vi "ActFollowTrajectoryCommon.vi"(10 "Trajectory":T4 {"States"."POSE"."ROTATION"."SIN" format="%13.4f"; "States"."POSE"."ROTATION"."COS" format="%13.4f"; "States"."POSE"."ROTATION"."VALUE" format="%13.4f"; "States"."POSE"."TRANSLATION"."Y" format="%14.3f"; "States"."POSE"."TRANSLATION"."X" format="%14.3f"; "TotalTImeSecs" format="%20.3f"}, 11 "FirstTime":bool) -> (0 "Done":bool, 1 "AngularSpeedDmd":dbl, 2 "YSpeedDmd":dbl, 3 "XSpeedDmd":dbl)   [LabVIEW 2020]
uses:
  <vilib>/Rock Robotics/WPI/ThirdParty/JAS_Junk/TrajLib/Trajectory_Library.lvlib
  <vilib>/Rock Robotics/WPI/ThirdParty/JAS_Junk/TrajLib/TypeDef/TRANSLATION2D.ctl
  <vilib>/Rock Robotics/WPI/ThirdParty/JAS_Junk/TrajLib/TypeDef/ROTATION2D.ctl
  <vilib>/Rock Robotics/WPI/ThirdParty/JAS_Junk/TrajLib/TypeDef/POSE2D.ctl
  <vilib>/Rock Robotics/WPI/ThirdParty/JAS_Junk/TrajLib/TypeDef/TRAJ_STATE.ctl
  <vilib>/Rock Robotics/WPI/ThirdParty/JAS_Junk/TrajLib/TypeDef/TRAJECTORY.ctl
panel:
  in  "currentPose":T1={"TRANSLATION"={"X"=0.0, "Y"=0.0}, "ROTATION"={"VALUE"=0.0, "COS"=1.0, "SIN"=0.0}} {"ROTATION"."SIN" format="%13.4f"; "ROTATION"."COS" format="%13.4f"; "ROTATION"."VALUE" format="%13.4f"; "TRANSLATION"."Y" format="%14.3f"; "TRANSLATION"."X" format="%14.3f"}
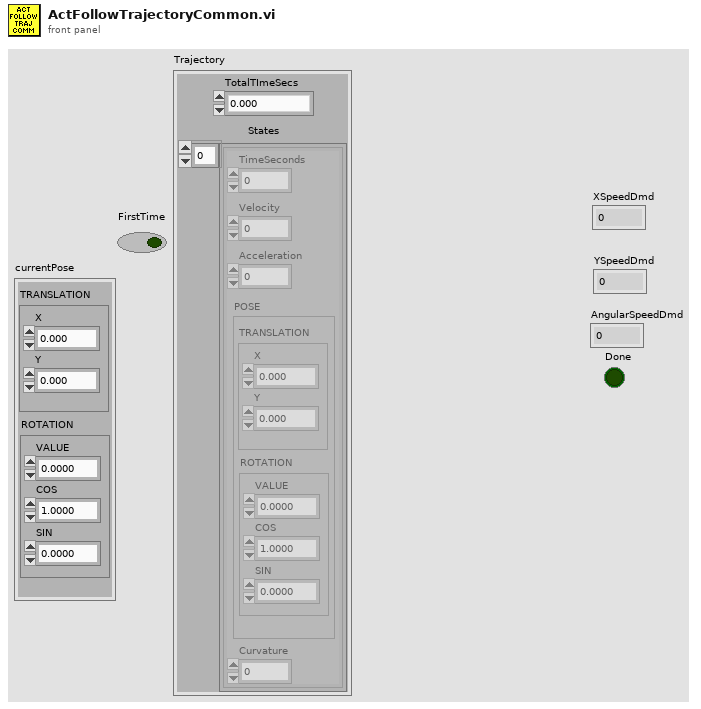
[diagram p1: front panel]
types:
  T1 = typedef "Trajectory_Library.lvlib/POSE2D.ctl" = cluster{"TRANSLATION":T2, "ROTATION":T3}
  T2 = typedef "Trajectory_Library.lvlib/TRANSLATION2D.ctl" = cluster{"X":dbl, "Y":dbl}
  T3 = typedef "Trajectory_Library.lvlib/ROTATION2D.ctl" = cluster{"VALUE":dbl, "COS":dbl, "SIN":dbl}
  T4 = typedef "Trajectory_Library.lvlib/TRAJECTORY.ctl" = cluster{"TotalTImeSecs":dbl, "States":T5[]}
  T5 = typedef "Trajectory_Library.lvlib/TRAJ_STATE.ctl" = cluster{"TimeSeconds":dbl, "Velocity":dbl, "Acceleration":dbl, "POSE":T1, "Curvature":dbl}
  T6 = typedef "Trajectory_Library.lvlib/PID_TUNING.ctl" = cluster{"Kp":dbl, "Ki":dbl, "Kd":dbl, "MaximumIntegral":dbl, "MinimumIntegral":dbl}
  T7 = typedef "Trajectory_Library.lvlib/PROFILED_PID_CONTROLLER.ctl" = cluster{"Controller":T8, "Goal":T9, "Setpoint":T9, "Constraint":T10}
  T8 = typedef "Trajectory_Library.lvlib/PID_CONTROLLER.ctl" = cluster{"Kp":dbl, "Ki":dbl, "Kd":dbl, "Period":dbl, "Max_Integral":dbl, "Min_Integral":dbl, "Max_Input":dbl, "Min_Input":dbl, "Continuous":bool, "PositionError":dbl, "VelocityError":dbl, "PrevError":dbl, "TotalError":dbl, "PositionTolerance":dbl, "VelocityTolerance":dbl, "SetPoint":dbl, "Kf":dbl, "Prev_Deriv":dbl, "Prev_Deriv 2":dbl, "DerivativeFilter":bool, "Min_Output":dbl, "Max_Output":dbl, "Prev_F_P":dbl, "Prev_F_P_2":dbl, "AntiWindupActive":bool, "Measurement":dbl}
  T9 = typedef "Trajectory_Library.lvlib/TRAPEZOID_PROFILE_STATE.ctl" = cluster{"Position":dbl, "Velocity":dbl}
  T10 = typedef "Trajectory_Library.lvlib/TRAPEZOID_PROFILE_CONSTRAINT.ctl" = cluster{"MaxVelocity":dbl, "MaxAcceleration":dbl}
  T11 = typedef "Trajectory_Library.lvlib/CHASSIS_SPEEDS.ctl" = cluster{"vX":dbl, "vY":dbl, "vOmega":dbl}
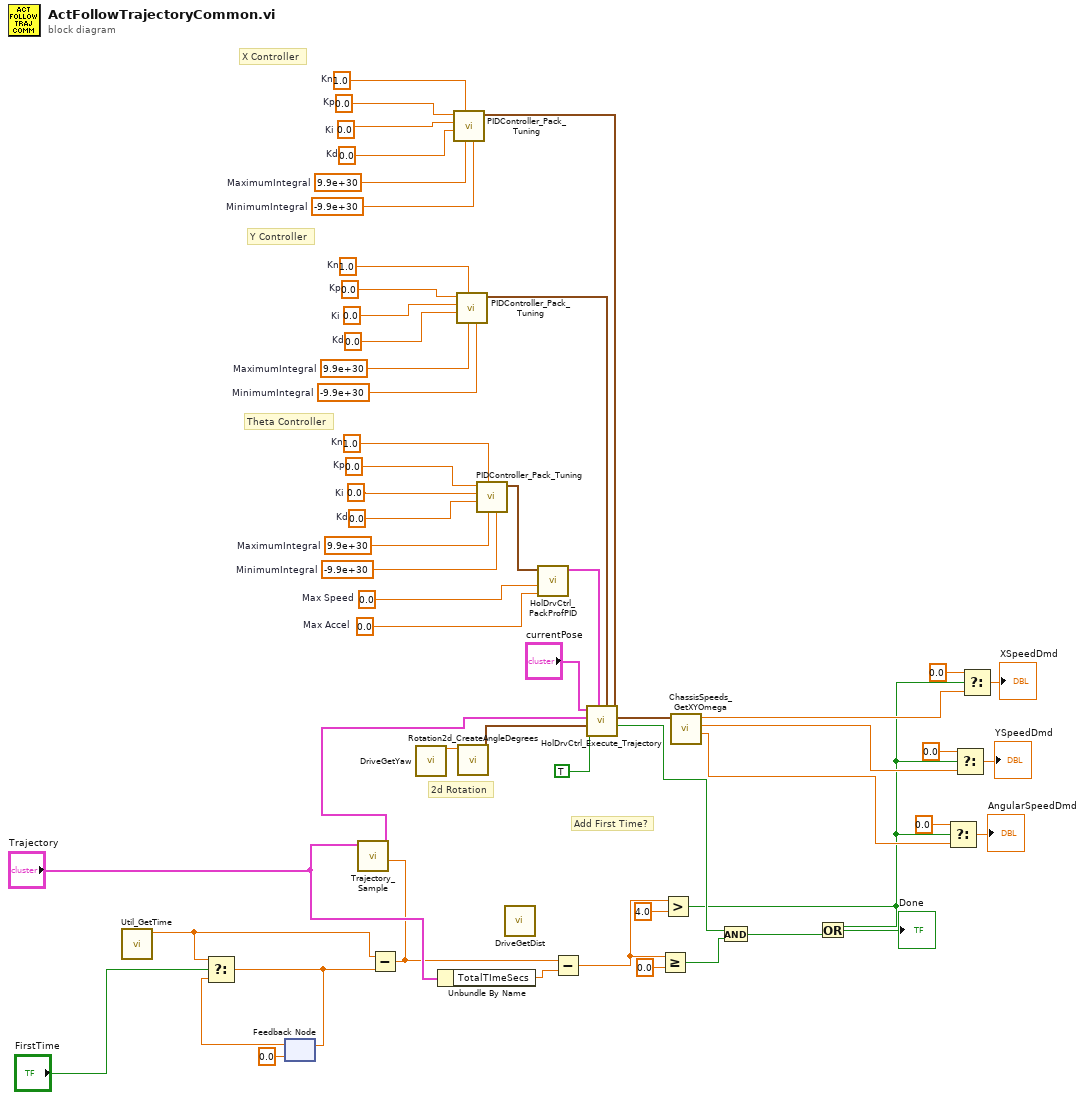
[diagram p0: block diagram]
diagram:
  w22 = 1.0  # Kn
  w25 = 0.0  # Kp
  w34 = 0.0  # Ki
  w35 = 0.0  # Kd
  w36 = 9.9e+30  # MaximumIntegral
  w37 = -9.9e+30  # MinimumIntegral
  w20 = 1.0  # Kn
  w23 = 0.0  # Kp
  w26 = 0.0  # Ki
  w27 = 0.0  # Kd
  w28 = 9.9e+30  # MaximumIntegral
  w29 = -9.9e+30  # MinimumIntegral
  w21 = 1.0  # Kn
  w24 = 0.0  # Kp
  w30 = 0.0  # Ki
  w31 = 0.0  # Kd
  w32 = 9.9e+30  # MaximumIntegral
  w33 = -9.9e+30  # MinimumIntegral
  w19 = 0.0  # Max Accel
  w18 = 0.0  # Max Speed
  # "Add First Time?"
  # "2d Rotation"
  # "Theta Controller"
  # "Y Controller"
  # "X Controller"
  n1 = call <vilib>:"Util_GetTime.vi"() -> ("FPGA_Time_Seconds"=w53:dbl)  [unwired: 9 in, 2 out]
  n2 = feedback #1(0.0) -> (w55:dbl)
  n3 = Select(t=w53, s="FirstTime", f=w55) -> (s? t:f=w52:dbl)
  n4 = feedback-in #1(w52) -> ()
  n5 = Subtract(x=w53, y=w52) -> (x-y=w49:dbl)
  n6 = call <vilib>:"Trajectory_Sample.vi"("Time"=w49, "InputTRAJECTORY"="Trajectory") -> ("OutputTRAJ_STATE"=w12:T5)  [unwired: 9 in]
  n7 = call "DriveGetYaw.vi"() -> ("Yaw"=w11:dbl)  [unwired: 11 in]
  n8 = Unbundle By Name("Trajectory") -> ("TotalTImeSecs"=w48:dbl)
  n9 = call <vilib>:"PIDController_Pack_Tuning.vi"("MinimumIntegral"=w29, "MaximumIntegral"=w28, "Kn"=w20, "Kd"=w27, "Ki"=w26, "Kp"=w23) -> ("PID Tuning"=w14:T6)  [unwired: 5 in]
  n10 = call <vilib>:"PIDController_Pack_Tuning.vi"("MinimumIntegral"=w33, "MaximumIntegral"=w32, "Kn"=w21, "Kd"=w31, "Ki"=w30, "Kp"=w24) -> ("PID Tuning"=w15:T6)  [unwired: 5 in]
  n11 = call <vilib>:"Rotation2d_CreateAngleDegrees.vi"("Angle_Degrees"=w11) -> ("ROTATION"=w10:T3)  [unwired: 10 in]
  n12 = call <vilib>:"PIDController_Pack_Tuning.vi"("MinimumIntegral"=w37, "MaximumIntegral"=w36, "Kn"=w22, "Kd"=w35, "Ki"=w34, "Kp"=w25) -> ("PID Tuning"=w17:T6)  [unwired: 5 in]
  n13 = call "DriveGetDist.vi"() -> ()  [unwired: 11 in, 1 out]
  n14 = call <vilib>:"HolDrvCtrl_PackProfPID.vi"("Max Accel"=w19, "Max Speed"=w18, "Theta PID Tuning"=w17) -> ("Theta PID CONTROLLER"=w16:T7)  [unwired: 8 in]
  n15 = Subtract(x=w49, y=w48) -> (x-y=w41:dbl)
  n16 = call <vilib>:"HolDrvCtrl_Execute_Trajectory.vi"("X PID Tuning"=w14, "Y PID Tuning"=w15, "thetaProfiledPID_CTRL"=w16, "Enable"=TRUE, "angleRef"=w10, "desiredTrajState"=w12, "currentPose"="currentPose") -> ("AtReference"=w8:bool, "calcChassisSpeed"=w7:T11)  [unwired: 2 in, 1 out]
  n17 = Greater Or Equal?(x=w41, y=0.0) -> (x >= y?=w40:bool)
  n18 = Greater?(x=w41, y=4.0) -> (0:w1:bool)
  n19 = call <vilib>:"ChassisSpeeds_GetXYOmega.vi"("CHASSIS"=w7) -> ("vAngular"=w2:dbl, "vY"=w3:dbl, "vX"=w4:dbl)  [unwired: 8 in]
  n20 = And(x=w8, y=w40) -> (x .and. y?=w46:bool)
  n21 = Or(x=w1, y=w46) -> (x .or. y?=→"Done":bool)
  n22 = Select(t=0.0, s=w1, f=w2) -> (s? t:f=→"AngularSpeedDmd":dbl)
  n23 = Select(t=0.0, s=w1, f=w3) -> (s? t:f=→"YSpeedDmd":dbl)
  n24 = Select(t=0.0, s=w1, f=w4) -> (s? t:f=→"XSpeedDmd":dbl)
